vi "Parse.vi"(8 "Error In":errorcluster, 11 "object in":refnum<class "2022_7.lvclass">) -> (0 "Error Out":errorcluster, 3 "object out":refnum<class "2022_7.lvclass">)   [LabVIEW 2020, in "2022_7.lvclass"]
uses:
  2022_7.lvclass
  2022_7.lvclass/2022_7.ctl
panel:
  out "CMDs":cluster{"CMDS":string[], "Return":string[]}[](array[cluster])
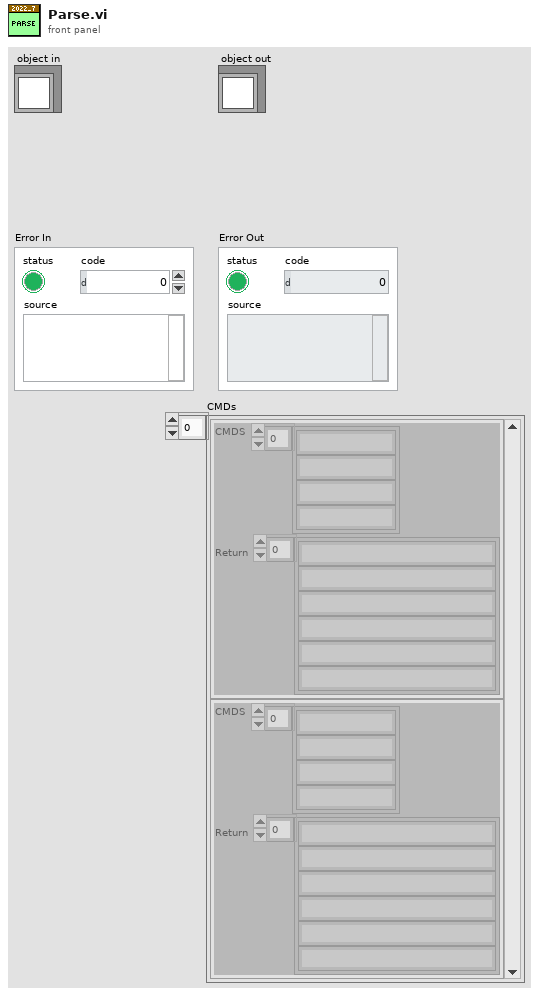
[diagram p1: front panel]
types:
  T1 = map{string[], cluster{"Folders":string[], "Files":cluster{"Name":string, "Size":i32}[]}}
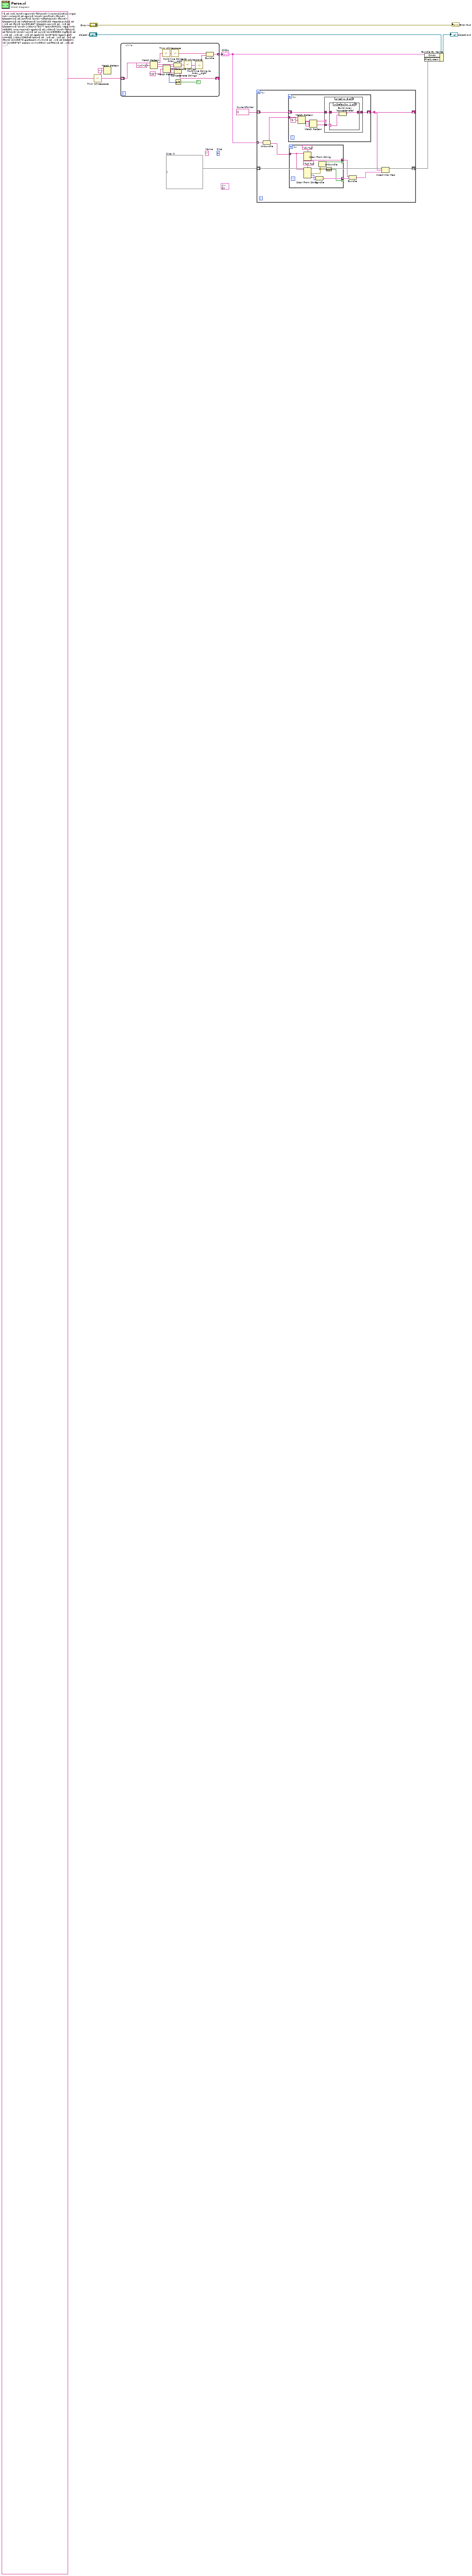
[diagram p0: block diagram]
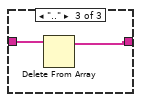
[diagram p5: hidden frame]
diagram:
  (unwired) cluster{"Name":string, "Size":i32} {"Name"="", "Size"=0} ("Cluster")
  (unwired) 0  # Size
  (unwired) ""  # Name
  w2 = T1 {}  # Size: 0
  w3 = string[] []  # CurrentFolder
  n1 = call <vilib>:"Trim Whitespace.vi"("string"="$ cd /\n$ ls\ndir cgw\ndir fbhz\ndir lvrzvt\n224312 vngq\ndir vwlps\n$ cd cgw\n$ ls\ndir jpmf\ndir rfb\ndir tjtccqtm\n$ cd jpmf\n$ ls\ndir ncfcchsz\ndir rfb\ndir tjtccqtm\n$ cd ncfcchsz\n$ ls\n205103 ntpprbt.pvt\n$ cd ..\n$ cd rfb\n$ ls\n331667 tjtccqtm.qzv\n$ cd ..\n$ cd tjtccqtm\n$ ls\ndir jvbb\n175277 tpc\n304201 vtgzj.hnb\n69381 wnq.npz\ndir zgpb\n$ cd jvbb\n$ ls\ndir fbhz\n$ cd fbhz\n$ ls\ndir wjj\n$ cd wjj\n$ ls\n255580 mgft\n$ cd ..\n$ cd ..\n$ cd ..\n$ cd zgpb\n$ ls\n57622 bgpm.gqf\n44482 jvbb\n156048 tpc\n$ cd ..\n$ cd ..\n$ cd ..\n$ cd rfb\n$ ls\n25370 gjptbqsm.mvm\n$ cd ..\n$ cd tjtccqtm\n$ ls\n359767 pcpqw.wvn\n9514 wplftrb\n$ cd ..\n$ cd ..\n$ cd fbhz\n$ ls\ndir fbhz\n328535 fbhz.fbd\n51958 fbhz.fbp\n37508 fcjgf.crj\ndir llfdghs\ndir ncfcchsz\n222206 srvhswd.mcg\ndir tbnq\n62795 vtgzj.hnb\ndir zhj\n$ cd fbhz\n$ ls\n363951 psm.lsv\n182275 sssdht.pqt\n44558 zvntd.hvr\n$ cd ..\n$ cd llfdghs\n$ ls\n126845 flg\ndir hsz\ndir mlvl\n199117 mzz.pbj\n141875 srvhswd.mcg\ndir tvtqs\n309288 wrbrmh\n$ cd hsz\n$ ls\ndir fbhz\n72585 mwlqg.rfg\n265089 ncfcchsz.cgj\ndir qsvh\n202721 vtgzj.hnb\n$ cd fbhz\n$ ls\n163444 nsrgjtl.dts\n$ cd ..\n$ cd qsvh\n$ ls\n260300 srvhswd.mcg\ndir tjtccqtm\n$ cd tjtccqtm\n$ ls\n311932 dhcmbc.ljq\n$ cd ..\n$ cd ..\n$ cd ..\n$ cd mlvl\n$ ls\n55902 rfb.jnd\n$ cd ..\n$ cd tvtqs\n$ ls\ndir fbhz\ndir hgr\ndir njvsjmmj\ndir tjtccqtm\n356368 tpc\ndir vgj\n$ cd fbhz\n$ ls\n196969 ncfcchsz.tfn\n176294 wzfchcvz.wwv\n$ cd ..\n$ cd hgr\n$ ls\ndir tjtccqtm\n$ cd tjtccqtm\n$ ls\n360282 vtgzj.hnb\n$ cd ..\n$ cd ..\n$ cd njvsjmmj\n$ ls\ndir gbrjnrh\n$ cd gbrjnrh\n$ ls\n270925 psm.lsv\n$ cd ..\n$ cd ..\n$ cd tjtccqtm\n$ ls\ndir nlqt\ndir tjtccqtm\n47866 vtgzj.hnb\n144250 zdg.brf\n$ cd nlqt\n$ ls\n49935 tpc\n$ cd ..\n$ cd tjtccqtm\n$ ls\n178987 sgpdvcf\n$ cd ..\n$ cd ..\n$ cd vgj\n$ ls\n213820 mcbph.srq\n$ cd ..\n$ cd ..\n$ cd ..\n$ cd ncfcchsz\n$ ls\n267915 fbhz\ndir tjtccqtm\n205385 zghlv.mtv\n$ cd tjtccqtm\n$ ls\n334824 ptbdgpn.wnz\n$ cd ..\n$ cd ..\n$ cd tbnq\n$ ls\n138692 dzwgs\n70126 gjps.vbz\ndir jvbb\ndir nzl\n196653 rsshtl.qlg\n110016 srvhswd.mcg\n217737 vngq\n$ cd jvbb\n$ ls\ndir wshhs\ndir ztrb\n$ cd wshhs\n$ ls\ndir bpcv\n285906 ntptv.hld\n182940 rfb.wfd\n24187 wgfmq\n$ cd bpcv\n$ ls\n108995 ncfcchsz.rmg\n304028 srvhswd.mcg\n$ cd ..\n$ cd ..\n$ cd ztrb\n$ ls\n88425 pfzbdqmw\n$ cd ..\n$ cd ..\n$ cd nzl\n$ ls\ndir fbhz\ndir jzvvr\ndir mghww\n131115 qcpdd.jfb\n208300 rqhtgdf.rqf\ndir tnfg\n$ cd fbhz\n$ ls\n317958 fbhz.pws\n$ cd ..\n$ cd jzvvr\n$ ls\n292945 dnqfmf.cwg\n8055 mwtrbv.sfm\n119001 rfb\ndir srgrvcm\n214676 srvhswd.mcg\n$ cd srgrvcm\n$ ls\ndir cfwmvbjq\ndir dqwwtrr\n102903 grhqhm.bhm\n360122 qmgtr.qmn\ndir tjtccqtm\n$ cd cfwmvbjq\n$ ls\n91385 vtgzj.hnb\n$ cd ..\n$ cd dqwwtrr\n$ ls\n151683 htg.ncm\n178927 vngq\n236079 vtgzj.hnb\n$ cd ..\n$ cd tjtccqtm\n$ ls\n334582 psm.lsv\n$ cd ..\n$ cd ..\n$ cd ..\n$ cd mghww\n$ ls\n48114 msvbqh\n$ cd ..\n$ cd tnfg\n$ ls\n172920 jhn.ghz\n$ cd ..\n$ cd ..\n$ cd ..\n$ cd zhj\n$ ls\ndir dqzgfcd\ndir jvbb\ndir ncnhjjs\n$ cd dqzgfcd\n$ ls\ndir ppmbn\ndir rfb\ndir srlvzvr\n225107 srvhswd.mcg\n353094 vngq\ndir vtdvdgdv\n297817 vtgzj.hnb\ndir vwhnlp\ndir wsmvrf\n$ cd ppmbn\n$ ls\n6037 vngq\n$ cd ..\n$ cd rfb\n$ ls\n293304 nzhchfrv.nst\n194726 rfb.gfs\n287537 tpc\n137637 vtgzj.hnb\ndir wdm\n$ cd wdm\n$ ls\n61473 psm.lsv\n152521 srvhswd.mcg\n$ cd ..\n$ cd ..\n$ cd srlvzvr\n$ ls\ndir dlp\n274123 whc.cjc\n$ cd dlp\n$ ls\ndir rfpgt\n$ cd rfpgt\n$ ls\n281038 jvbb.mnq\n312481 mmjcgss\n186883 vdpq.qzn\n194336 wvjrhdq.llv\n$ cd ..\n$ cd ..\n$ cd ..\n$ cd vtdvdgdv\n$ ls\ndir rfb\ndir tjtccqtm\n$ cd rfb\n$ ls\n196456 dprdjqnp.wqc\n67720 psm.lsv\n820 rfb.jrh\n170351 tpc\n$ cd ..\n$ cd tjtccqtm\n$ ls\n269007 bsrvltnf\n$ cd ..\n$ cd ..\n$ cd vwhnlp\n$ ls\ndir fbhz\n30697 ncfcchsz.dlh\ndir rfb\ndir tjtccqtm\n185165 vtgzj.hnb\n$ cd fbhz\n$ ls\ndir dstmnnd\n65237 dvhhwv.zqz\n156937 gtbzgp\ndir jvbb\ndir ncfcchsz\ndir wdpqfl\n$ cd dstmnnd\n$ ls\n334642 grbvbw\ndir jvbb\n$ cd jvbb\n$ ls\n187235 bgrhrn.wmt\n$ cd ..\n$ cd ..\n$ cd jvbb\n$ ls\ndir dcszm\n280304 fbhz.bfq\n161981 jrgqlf\ndir mvcfwwlm\n194182 psm.lsv\ndir rfb\n40787 zrscw\n$ cd dcszm\n$ ls\n178161 gfc.nss\n$ cd ..\n$ cd mvcfwwlm\n$ ls\n284005 hvzzlc\n$ cd ..\n$ cd rfb\n$ ls\n295068 fbhz.ccj\ndir jvbb\n73713 mqs\ndir ncfcchsz\n99417 psps.pnc\ndir rhmmtvv\n$ cd jvbb\n$ ls\n62151 hlblqv.cbq\n318565 jvbb.rgv\n230913 ppq.chd\n$ cd ..\n$ cd ncfcchsz\n$ ls\n133380 srvhswd.mcg\n$ cd ..\n$ cd rhmmtvv\n$ ls\n270217 qms.zrf\n$ cd ..\n$ cd ..\n$ cd ..\n$ cd ncfcchsz\n$ ls\ndir bzpz\ndir fmhdlm\ndir wqctddqc\n$ cd bzpz\n$ ls\n270136 tpc\n271633 vtgzj.hnb\n$ cd ..\n$ cd fmhdlm\n$ ls\n273720 mgf.pdm\n23453 rfb.lvs\n49685 tld.vbh\n$ cd ..\n$ cd wqctddqc\n$ ls\ndir ncfcchsz\n$ cd ncfcchsz\n$ ls\n111237 vqvs\n$ cd ..\n$ cd ..\n$ cd ..\n$ cd wdpqfl\n$ ls\ndir fmrclsn\n258435 fzgtz.bhg\ndir mwwmbpgr\ndir nsf\ndir tfpqqjw\n118118 tjtccqtm\n219688 tjtccqtm.tst\n$ cd fmrclsn\n$ ls\n271116 gzbqm.tnj\n216909 jvbb\n167454 qnfdzw.slr\n252140 tsrzcnjb\n$ cd ..\n$ cd mwwmbpgr\n$ ls\ndir jvbb\ndir rqfqbw\n$ cd jvbb\n$ ls\n44631 tjtccqtm\n$ cd ..\n$ cd rqfqbw\n$ ls\ndir cqpwhrtp\n$ cd cqpwhrtp\n$ ls\n305787 vjndql.qqv\n$ cd ..\n$ cd ..\n$ cd ..\n$ cd nsf\n$ ls\n211811 ggztzqp\n69628 vtgzj.hnb\n$ cd ..\n$ cd tfpqqjw\n$ ls\n295011 ncfcchsz.dnn\n88554 psm.lsv\n$ cd ..\n$ cd ..\n$ cd ..\n$ cd rfb\n$ ls\n51633 ncfcchsz\n318667 psm.lsv\n49231 qnsldrn\n240239 sdcmgc.gdt\ndir tgcr\n121575 vtgzj.hnb\n$ cd tgcr\n$ ls\n198742 rfb.nsl\n$ cd ..\n$ cd ..\n$ cd tjtccqtm\n$ ls\ndir vnwpw\n$ cd vnwpw\n$ ls\n338543 htwmhv\n18782 lvwjtn.dcz\n212005 ncfcchsz\ndir rfb\ndir tjhvvl\n95069 vtgzj.hnb\n117084 wsfvhn\n$ cd rfb\n$ ls\n89621 fbhz.vnm\n$ cd ..\n$ cd tjhvvl\n$ ls\n262643 clmfhnct.wrt\ndir fbhz\n101520 ncfcchsz\n169089 vtf.bmc\n72983 zgjw.wpn\n74431 zlwvcwn.gzf\n$ cd fbhz\n$ ls\n213519 zpvhg\n$ cd ..\n$ cd ..\n$ cd ..\n$ cd ..\n$ cd ..\n$ cd wsmvrf\n$ ls\ndir ccbw\ndir nqjpdlc\n253007 rfb\ndir sjgjgwb\ndir zprqg\n$ cd ccbw\n$ ls\ndir crjsgdv\ndir dthrqpvv\ndir ncfcchsz\ndir ppqhd\ndir tjtccqtm\ndir ztsmqn\n$ cd crjsgdv\n$ ls\ndir jgstsj\n169620 vngq\n$ cd jgstsj\n$ ls\n251288 vtgzj.hnb\n$ cd ..\n$ cd ..\n$ cd dthrqpvv\n$ ls\n234510 fldrtqh.cbq\n$ cd ..\n$ cd ncfcchsz\n$ ls\n177247 dbt.fsb\n$ cd ..\n$ cd ppqhd\n$ ls\n21458 psm.lsv\n20155 tjtccqtm.rsn\n$ cd ..\n$ cd tjtccqtm\n$ ls\n71907 psm.lsv\n$ cd ..\n$ cd ztsmqn\n$ ls\n124096 gjzgbrj.sjn\n$ cd ..\n$ cd ..\n$ cd nqjpdlc\n$ ls\ndir jvbb\ndir ltwl\n143570 lwcgls.qvp\n$ cd jvbb\n$ ls\n266605 qvwfhw.qvh\n$ cd ..\n$ cd ltwl\n$ ls\ndir lrgjbbn\n$ cd lrgjbbn\n$ ls\n68291 tjtccqtm.rlr\n$ cd ..\n$ cd ..\n$ cd ..\n$ cd sjgjgwb\n$ ls\n265194 ddv\ndir ghqtfhcz\ndir jwzmtqff\n15930 mzgtdwsg\n$ cd ghqtfhcz\n$ ls\ndir gtlfvjpg\n$ cd gtlfvjpg\n$ ls\ndir vwz\n$ cd vwz\n$ ls\n252002 tpc\n$ cd ..\n$ cd ..\n$ cd ..\n$ cd jwzmtqff\n$ ls\n238465 gsr.mrj\n332865 gzfcfqn.lbd\n$ cd ..\n$ cd ..\n$ cd zprqg\n$ ls\n148532 nzjwc\n179858 plznjhb\n70176 tpc\n$ cd ..\n$ cd ..\n$ cd ..\n$ cd jvbb\n$ ls\ndir bnllsz\ndir cqdr\n293380 hrszhbzc.rrq\n253762 jvbb\ndir jwn\n251152 lchdqwvg\ndir lrh\ndir nfbhj\ndir nnflrw\ndir rfb\n293144 srvhswd.mcg\n104936 vtgzj.hnb\n$ cd bnllsz\n$ ls\n216397 vngq\n$ cd ..\n$ cd cqdr\n$ ls\n272746 psm.lsv\n81840 tpc\n$ cd ..\n$ cd jwn\n$ ls\n224049 fhl.mrh\n342246 tpc\n233666 zmbg\n$ cd ..\n$ cd lrh\n$ ls\n139676 mcdv\n$ cd ..\n$ cd nfbhj\n$ ls\n49779 rfb.tnm\n$ cd ..\n$ cd nnflrw\n$ ls\n56516 hgtjdb\n79167 psm.lsv\n$ cd ..\n$ cd rfb\n$ ls\n65765 mcdv\n$ cd ..\n$ cd ..\n$ cd ncnhjjs\n$ ls\ndir jvbb\n276470 ncfcchsz\n273860 vngq\n$ cd jvbb\n$ ls\n9420 psmrjhmp.dfj\n$ cd ..\n$ cd ..\n$ cd ..\n$ cd ..\n$ cd lvrzvt\n$ ls\n26201 ncfcchsz.zrn\n267647 ncppww\ndir qzddwnm\n345874 tpc\n115177 vtgzj.hnb\ndir zzwqlz\n$ cd qzddwnm\n$ ls\n214814 psm.lsv\n$ cd ..\n$ cd zzwqlz\n$ ls\n181990 pcz.ctb\n258280 tjtccqtm\n37664 vtgzj.hnb\n$ cd ..\n$ cd ..\n$ cd vwlps\n$ ls\ndir fbhz\ndir jvbb\n347635 psm.lsv\n101891 pzzt.prc\ndir rfb\ndir tjtccqtm\n322963 tjtccqtm.swf\n$ cd fbhz\n$ ls\ndir fbhz\n$ cd fbhz\n$ ls\ndir mnnzbnl\n115 zhgrzjt.hlq\n$ cd mnnzbnl\n$ ls\n624 vngq\n$ cd ..\n$ cd ..\n$ cd ..\n$ cd jvbb\n$ ls\n149547 jtng.qfh\n84714 wqqnqpc.crj\n$ cd ..\n$ cd rfb\n$ ls\ndir ddcjgrdb\n26416 jvbb.nbg\ndir lwjvv\ndir mtzbmlnp\ndir nsq\n42884 pmzdjzmv\n305628 sgc\n109079 srvhswd.mcg\n303802 tpc\n$ cd ddcjgrdb\n$ ls\ndir jvbb\ndir rfb\n$ cd jvbb\n$ ls\n348073 jgwzvs\n$ cd ..\n$ cd rfb\n$ ls\ndir tjtccqtm\n119113 tpc\n$ cd tjtccqtm\n$ ls\n357579 rfb\n124868 srvhswd.mcg\n$ cd ..\n$ cd ..\n$ cd ..\n$ cd lwjvv\n$ ls\n212416 fbglfwjn\ndir hhjlvjds\n158555 tpc\ndir tvqng\n287589 vngq\ndir zcn\n$ cd hhjlvjds\n$ ls\n57297 przml.gfn\n173735 psm.lsv\n245882 srvhswd.mcg\n244645 tjtccqtm.gnh\n289149 vngq\ndir zmzj\n$ cd zmzj\n$ ls\n28824 vngq\n$ cd ..\n$ cd ..\n$ cd tvqng\n$ ls\n136988 fbhz.wnl\n$ cd ..\n$ cd zcn\n$ ls\ndir czczrddv\n$ cd czczrddv\n$ ls\n239586 zjwswstd.mdj\n$ cd ..\n$ cd ..\n$ cd ..\n$ cd mtzbmlnp\n$ ls\ndir fbhz\ndir jvbb\n231169 mnrbmhvt\ndir nhfsqbb\ndir sjmm\ndir ttsjtcc\n$ cd fbhz\n$ ls\ndir lhtc\ndir tjtccqtm\n9513 vtgzj.hnb\n$ cd lhtc\n$ ls\n100051 fbhz.cvg\n$ cd ..\n$ cd tjtccqtm\n$ ls\n193182 psm.lsv\n$ cd ..\n$ cd ..\n$ cd jvbb\n$ ls\n224879 hvswfzqc.zmc\ndir rfb\n202937 rflsltm.bcc\ndir tjtccqtm\n$ cd rfb\n$ ls\n238032 fbhz\ndir fgctrfr\n306802 jvbb\n225954 ncfcchsz.lcs\ndir tjtccqtm\n$ cd fgctrfr\n$ ls\ndir dqjrndw\n103974 jmmjds\n233363 mqr.zhm\n334730 psm.lsv\ndir rbbw\n281420 tjtccqtm\ndir zgrrdb\n$ cd dqjrndw\n$ ls\n295822 tpc\n$ cd ..\n$ cd rbbw\n$ ls\ndir hrwj\n$ cd hrwj\n$ ls\ndir zlhhnwrv\n$ cd zlhhnwrv\n$ ls\n168370 tjtccqtm.dnn\n$ cd ..\n$ cd ..\n$ cd ..\n$ cd zgrrdb\n$ ls\n84053 vtgzj.hnb\n$ cd ..\n$ cd ..\n$ cd tjtccqtm\n$ ls\n297111 jpnzcw.srg\n$ cd ..\n$ cd ..\n$ cd tjtccqtm\n$ ls\ndir jfmc\ndir qwrd\ndir tjtccqtm\n$ cd jfmc\n$ ls\ndir fbhz\ndir fjqnrb\ndir mpc\ndir ncfcchsz\n139767 vtgzj.hnb\n$ cd fbhz\n$ ls\ndir rfb\ndir tqmtbvb\n$ cd rfb\n$ ls\n304548 jhrjt\n$ cd ..\n$ cd tqmtbvb\n$ ls\n62368 vngq\n$ cd ..\n$ cd ..\n$ cd fjqnrb\n$ ls\ndir qdrmjmds\ndir rfb\ndir sdtdrmz\n$ cd qdrmjmds\n$ ls\ndir qscgv\ndir rfb\n$ cd qscgv\n$ ls\n173814 ncfcchsz.nch\n$ cd ..\n$ cd rfb\n$ ls\n1592 vtgzj.hnb\n$ cd ..\n$ cd ..\n$ cd rfb\n$ ls\n237598 dvbnmp.bcw\n$ cd ..\n$ cd sdtdrmz\n$ ls\n43253 sqdd\n$ cd ..\n$ cd ..\n$ cd mpc\n$ ls\ndir bdsnl\n$ cd bdsnl\n$ ls\n175855 psm.lsv\n$ cd ..\n$ cd ..\n$ cd ncfcchsz\n$ ls\ndir ctqnwzgn\ndir dddjjbrs\ndir nbnn\ndir tjtccqtm\n$ cd ctqnwzgn\n$ ls\n211637 ncfcchsz\n$ cd ..\n$ cd dddjjbrs\n$ ls\n160464 bjbdh.mtr\n139283 jjgblbjc.bvn\ndir lqpsr\n155029 szcpzjz.vtv\n$ cd lqpsr\n$ ls\n314159 mdzgl.jqd\n$ cd ..\n$ cd ..\n$ cd nbnn\n$ ls\n218457 tpc\n$ cd ..\n$ cd tjtccqtm\n$ ls\ndir rfb\n109587 tfw\ndir vqsjdd\n$ cd rfb\n$ ls\n240479 rblwfbn\n$ cd ..\n$ cd vqsjdd\n$ ls\n253970 srvhswd.mcg\n$ cd ..\n$ cd ..\n$ cd ..\n$ cd ..\n$ cd qwrd\n$ ls\ndir dgf\n$ cd dgf\n$ ls\n340237 fbsfq.mls\ndir tjtccqtm\ndir ttqnbdjn\n$ cd tjtccqtm\n$ ls\ndir msgtcp\n$ cd msgtcp\n$ ls\n245596 fbhz\n$ cd ..\n$ cd ..\n$ cd ttqnbdjn\n$ ls\ndir gvll\n$ cd gvll\n$ ls\ndir bhhzh\n$ cd bhhzh\n$ ls\n153339 wcqpmnb.slt\n$ cd ..\n$ cd ..\n$ cd ..\n$ cd ..\n$ cd ..\n$ cd tjtccqtm\n$ ls\ndir nzbzjpnl\n$ cd nzbzjpnl\n$ ls\n72123 dzpjf.wmb\n35136 ncfcchsz.qnz\n234519 vhq.vrr\n$ cd ..\n$ cd ..\n$ cd ..\n$ cd ..\n$ cd nhfsqbb\n$ ls\n109518 tqnct.jvf\n51666 vngq\n$ cd ..\n$ cd sjmm\n$ ls\n263022 psm.lsv\ndir qrpr\ndir rfb\n$ cd qrpr\n$ ls\n51657 tpc\n$ cd ..\n$ cd rfb\n$ ls\n185213 fllcngdc\n$ cd ..\n$ cd ..\n$ cd ttsjtcc\n$ ls\ndir fbhz\ndir tjbnz\n$ cd fbhz\n$ ls\n112216 slzn.jls\n$ cd ..\n$ cd tjbnz\n$ ls\n73261 fbhz.wtd\n$ cd ..\n$ cd ..\n$ cd ..\n$ cd nsq\n$ ls\n93689 srvhswd.mcg\n$ cd ..\n$ cd ..\n$ cd tjtccqtm\n$ ls\n232421 vngq\n" ("PuzzleInput")) -> ("trimmed string"=w6:string)  [unwired: 1 in]
  n2 = Match Pattern(string=w6, regular expression="") -> ()  [unwired: 1 in, 4 out]
  n3 = while {
    shift-right: [w13] -> _
    shift-left: w6 -> [w28]
    tunnel: [w16] -> w4 mode=indexing
    stop <- w11 continue-if-true
    n4 = Match Pattern(string=w28, regular expression="\\n[~$]") -> (before substring=w24:string, match substring=w21:string, after substring=w26:string)  [unwired: 1 in, 1 out]
    n5 = call <vilib>:"Trim Whitespace.vi"("string"=w24) -> ("trimmed string"=w22:string)  [unwired: 1 in]
    n6 = Match Pattern(string=w26, regular expression="\\$") -> (before substring=w20:string, match substring=w15:string, after substring=w14:string, offset past match=w12:i32)  [unwired: 1 in]
    n7 = call <userlib>:"Multi-line String to Array__ogtk.vi"("string"=w22) -> ("lines"=w23:string[])
    n8 = Concatenate Strings(w21, w20) -> (w19:string)
    n9 = Concatenate Strings(w15, w14) -> (w13:string)
    n10 = Greater Or Equal To 0?(x=w12) -> (x >= 0?=w11:bool)
    n11 = call <vilib>:"Trim Whitespace.vi"("string"=w19) -> ("trimmed string"=w18:string)  [unwired: 1 in]
    n12 = call <userlib>:"Multi-line String to Array__ogtk.vi"("string"=w18) -> ("lines"=w17:string[])
    n13 = Bundle("lines"=w23, "lines"=w17) -> (w16:cluster{"lines":string[], "lines":string[]})  [unwired: 1 in]
  }
  "CMDs" <- w4
  n14 = for {
    tunnel: w4 -> [w38] mode=indexing
    shift-right: [w34] -> _
    shift-left: w3 -> [w37]
    shift-right: [w29] -> w1
    shift-left: w2 -> [w35]
    n15 = Unbundle(w38) -> ("lines"=w36:string[], "lines"=w33:string[])
    n16 = for {
      shift-right: [w50] -> w34
      shift-left: w37 -> [w51]
      tunnel: w36 -> [w56] mode=indexing
      n17 = Match Pattern(string=w56, regular expression="$ ") -> (after substring=w54:string)  [unwired: 1 in, 3 out]
      n18 = Match Pattern(string=w54, regular expression=" ") -> (before substring=w52:string, after substring=w49:string)  [unwired: 1 in, 2 out]
      n19 = case shown="\"cd\"" w52 {
        tunnel: w51 -> [w57 w58 w59]
        tunnel: [w57 w58 w60] -> w50
        tunnel: w49 -> [_ _ w61]
        frame Default {
        }
        frame "ls" {
        }
        frame "cd" {
          n20 = case shown="Default" w61 {
            selector: w61 -> [w63 _ _]
            tunnel: [w62 _ w65] -> w60
            tunnel: w59 -> [w64 _ w66]
            frame Default {
              n21 = Build Array (concatenate)(w64, w63) -> (w62:string[])
            }
            frame "/" {
            }
            frame ".." {
              n22 = Delete From Array(array=w66) -> (array with subset deleted=w65:string[])  [unwired: 2 in, 1 out]
            }
          }
        }
      }
    }
    n23 = for {
      tunnel: w33 -> [w47] mode=indexing
      tunnel: [w45] -> w31 mode=indexing if=w39
      tunnel: [w42] -> w32 mode=indexing if=w41
      n24 = Scan From String(format string="dir %s", input string=w47) -> (output 1=w45:string)  [unwired: 3 in, 3 out]
      n25 = Scan From String(format string="%d %s", input string=w47) -> (error out=w40:errorcluster, output 1=w43:i32, output 2=w44:string)  [unwired: 4 in, 2 out]
      n26 = Bundle(w44, w43) -> (w42:cluster{string, i32})  [unwired: 1 in]
      n27 = Unbundle(w40) -> ("status"=w39:bool)  [unwired: 2 out]
      n28 = Not(x=w40) -> (.not. x?=w41:bool)
    }
    n29 = Bundle(w31, w32) -> (w30:cluster{string[], cluster{string, i32}[]})  [unwired: 1 in]
    n30 = Insert Into Map(map in=w35, key=w34, value=w30) -> (map out=w29:T1)  [unwired: 2 out]
  }
  n31 = Bundle By Name(cluster="object in", "Cmds"=w4, "FileSystem"=w1) -> (→"object out":refnum<class "2022_7.lvclass">)
  "Error Out" <- "Error In"
